vi "IMAQ FPGA Camera Link Pixel Bus to Vision Pixel Bus.vi"   [LabVIEW 2017]
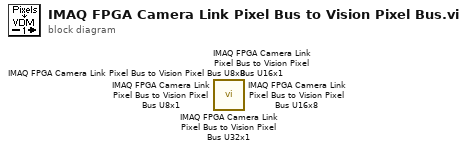
[diagram p0: block diagram]
diagram:
  n1 = call <vilib>:"IMAQ FPGA Camera Link Pixel Bus to Vision Pixel Bus U32x1.vi"() -> ()  [unwired: 9 in, 3 out]
  n2 = call <vilib>:"IMAQ FPGA Camera Link Pixel Bus to Vision Pixel Bus U16x1.vi"() -> ()  [unwired: 9 in, 3 out]
  n3 = call <vilib>:"IMAQ FPGA Camera Link Pixel Bus to Vision Pixel Bus U8x1.vi"() -> ()  [unwired: 9 in, 3 out]
  n4 = call <vilib>:"IMAQ FPGA Camera Link Pixel Bus to Vision Pixel Bus U16x8.vi"() -> ()  [unwired: 9 in, 3 out]
  n5 = call <vilib>:"IMAQ FPGA Camera Link Pixel Bus to Vision Pixel Bus U8x8.vi"() -> ()  [unwired: 9 in, 3 out]
